vi "DLL Library Path VIs.vi"() -> (0 "OCTNumerics":path, 1 "Alazar":path, 2 "GPU FFT amp amp phase diff":path, 7 "GPU FFT amp amp phase phase":path, 9 "GPU FFT amp amp":path, 10 "GPU FFT single amp phase":path, 11 "GPU FFT single amp":path)   [LabVIEW 2018]
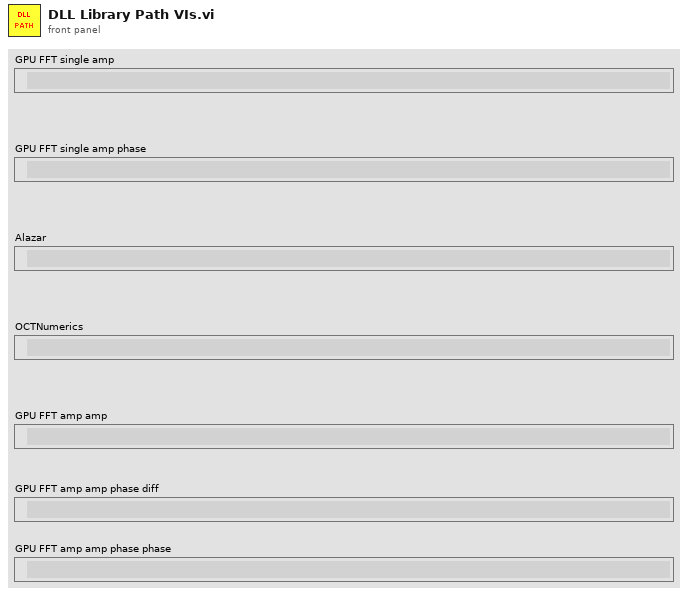
[diagram p1: front panel]
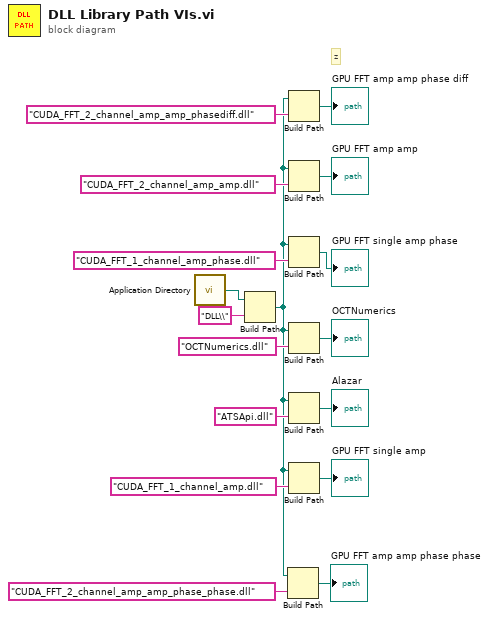
[diagram p0: block diagram]
diagram:
  # "z"
  n1 = call <vilib>:"Application Directory.vi"() -> ("Application Directory"=w17:path)
  n2 = Build Path(base path=w17, name or relative path="DLL\\") -> (appended path=w1:path)
  n3 = Build Path(base path=w1, name or relative path="CUDA_FFT_2_channel_amp_amp_phase_phase.dll") -> (appended path=→"GPU FFT amp amp phase phase":path)
  n4 = Build Path(base path=w1, name or relative path="CUDA_FFT_2_channel_amp_amp_phasediff.dll") -> (appended path=→"GPU FFT amp amp phase diff":path)
  n5 = Build Path(base path=w1, name or relative path="CUDA_FFT_2_channel_amp_amp.dll") -> (appended path=→"GPU FFT amp amp":path)
  n6 = Build Path(base path=w1, name or relative path="CUDA_FFT_1_channel_amp_phase.dll") -> (appended path=→"GPU FFT single amp phase":path)
  n7 = Build Path(base path=w1, name or relative path="OCTNumerics.dll") -> (appended path=→"OCTNumerics":path)
  n8 = Build Path(base path=w1, name or relative path="ATSApi.dll") -> (appended path=→"Alazar":path)
  n9 = Build Path(base path=w1, name or relative path="CUDA_FFT_1_channel_amp.dll") -> (appended path=→"GPU FFT single amp":path)
